vi "Class Implements Method.vi"(8 "error in (no error)":errorcluster, 10 "Method Name":string, 11 "Class Refnum":refnum<vi>) -> (0 "error out":errorcluster, 2 "Implements method?":bool, 3 "Class Refnum out":refnum<vi>)   [LabVIEW 2020, in "Choose Implementation Dialog.lvlib"]
uses:
  Choose Implementation Dialog.lvlib
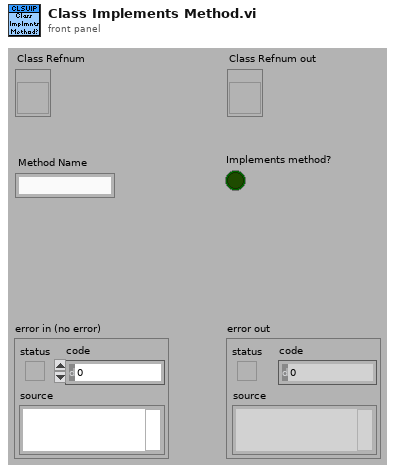
[diagram p1: front panel]
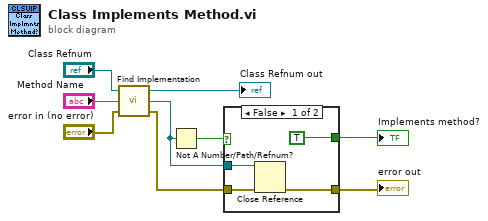
[diagram p0: block diagram]
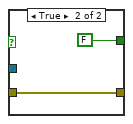
[diagram p2: hidden frame]
diagram:
  n1 = call "Find Implementation.vi"("error in"="error in (no error)", "Method Name"="Method Name", "Class in"="Class Refnum") -> ("error out"=w4:errorcluster, "VI"=w3:refnum<vi>, "Class out"=→"Class Refnum out":refnum<vi>)
  n2 = Not A Number/Path/Refnum?(number/path/refnum=w3) -> (NaN/Path/Refnum?=w2:bool)
  n3 = case shown="False" w2 {
    tunnel: [w13 w15] -> w5
    tunnel: w4 -> [w12 w15]
    tunnel: w3 -> [w11 _]
    tunnel: [TRUE FALSE] -> w1
    frame False {
      n4 = Close Reference(reference=w11, error in (no error)=w12) -> (error out=w13:errorcluster)
    }
    frame True {
    }
  }
  "error out" <- w5
  "Implements method?" <- w1
